vi "Data window -- tdms manage.vi"(7 "Data window action":T1, 8 "Length IN":i32, 9 "Start IN":i64, 11 "Data window IN":T2={"Start"=313333, "Length"=3333, "Channel numbers"=[0], "Channel names"=["freq", "Field"], "Group name"="p"}) -> (0 "Length OUT":i32, 1 "Start OUT":i64, 3 "Data window OUT":T2={"Start"=313333, "Length"=3333, "Channel numbers"=[0], "Channel names"=["freq", "Field"], "Group name"="p"})   [LabVIEW 2021]
uses:
  fft -- data win.ctl
  Data window -- tdms manage -- control.ctl
panel:
  # "OR"
  # "OR"
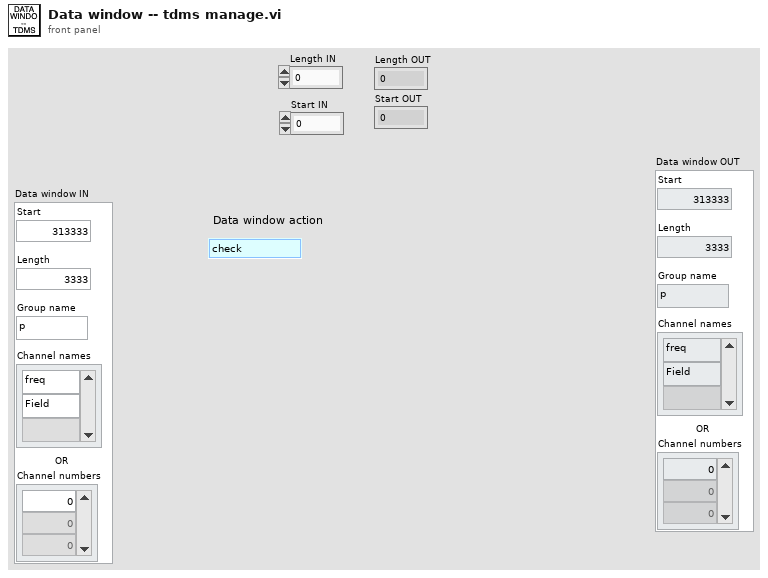
[diagram p1: front panel]
types:
  T1 = typedef "Data window -- tdms manage -- control.ctl" = enum16{"check", "set start&len", "set field channel", "set freq channel"}
  T2 = typedef "fft -- data win.ctl" = cluster{"Start":i64, "Length":i32, "Channel numbers":i64[], "Channel names":string[], "Group name":string}
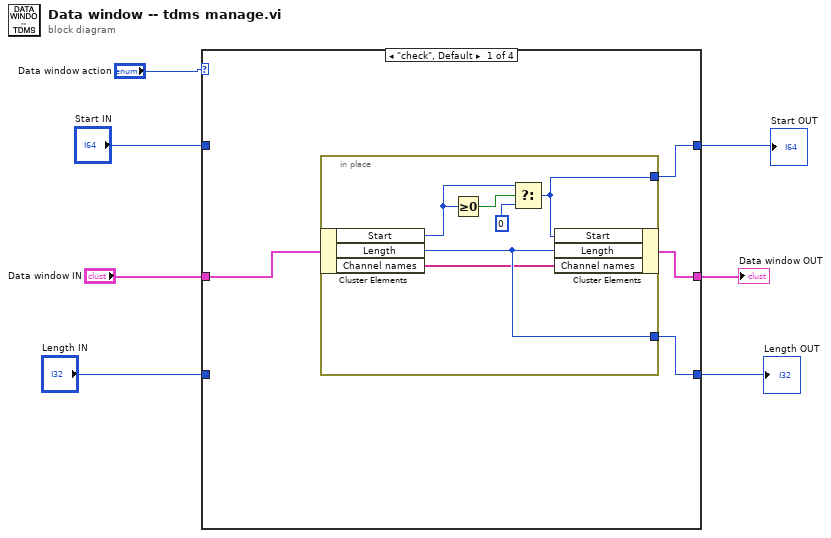
[diagram p0: block diagram]
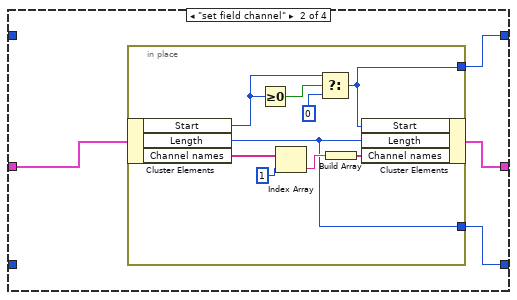
[diagram p2: hidden frame]
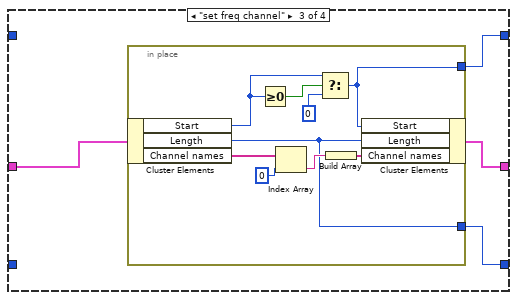
[diagram p3: hidden frame]
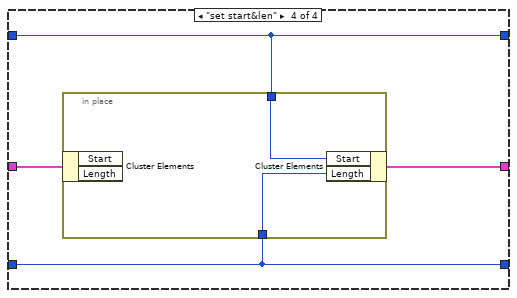
[diagram p4: hidden frame]
diagram:
  n1 = case shown="\"check\", Default" "Data window action" {
    tunnel: "Data window IN" -> [w11 w21 w34 w44]
    tunnel: [w10 w20 w33 w47] -> w5
    tunnel: [w9 w19 w32 w45] -> w4
    tunnel: [w8 w18 w31 w46] -> w3
    tunnel: "Start IN" -> [_ _ _ w46]
    tunnel: "Length IN" -> [_ _ _ w45]
    frame "check", Default {
      n2 = in-place {
        in-place-border: [w14] -> w9
        in-place-border: [w13] -> w8
        n3 = in-place-cluster #1(w11) -> ("Start"=w15:i64, "Length"=w14:i32, "Channel names"=w12:string[])
        n4 = Greater Or Equal To 0?(x=w15) -> (x >= 0?=w17:bool)
        n5 = Select(t=w15, s=w17, f=i64 0 ("Start")) -> (s? t:f=w13:i64)
        n6 = in-place-cluster #1("Start"=w13, "Length"=w14, "Channel names"=w12) -> (w10:T2)
      }
    }
    frame "set field channel" {
      n7 = in-place {
        in-place-border: [w23] -> w19
        in-place-border: [w22] -> w18
        n8 = in-place-cluster #2(w21) -> ("Start"=w24:i64, "Length"=w23:i32, "Channel names"=w28:string[])
        n9 = Greater Or Equal To 0?(x=w24) -> (x >= 0?=w30:bool)
        n10 = Index Array(array=w28, index=1) -> (element=w27:string)
        n11 = Select(t=w24, s=w30, f=i64 0 ("Start")) -> (s? t:f=w22:i64)
        n12 = Build Array(w27) -> (w26:string[])
        n13 = in-place-cluster #2("Start"=w22, "Length"=w23, "Channel names"=w26) -> (w20:T2)
      }
    }
    frame "set freq channel" {
      n14 = in-place {
        in-place-border: [w36] -> w32
        in-place-border: [w35] -> w31
        n15 = in-place-cluster #3(w34) -> ("Start"=w37:i64, "Length"=w36:i32, "Channel names"=w41:string[])
        n16 = Greater Or Equal To 0?(x=w37) -> (x >= 0?=w43:bool)
        n17 = Index Array(array=w41, index=0) -> (element=w40:string)
        n18 = Select(t=w37, s=w43, f=i64 0 ("Start")) -> (s? t:f=w35:i64)
        n19 = Build Array(w40) -> (w39:string[])
        n20 = in-place-cluster #3("Start"=w35, "Length"=w36, "Channel names"=w39) -> (w33:T2)
      }
    }
    frame "set start&len" {
      n21 = in-place {
        in-place-border: w46 -> [w49]
        in-place-border: w45 -> [w48]
        n22 = in-place-cluster #4(w44) -> ()  [unwired: 2 out]
        n23 = in-place-cluster #4("Start"=w49, "Length"=w48) -> (w47:T2)
      }
    }
  }
  "Data window OUT" <- w5
  "Length OUT" <- w4
  "Start OUT" <- w3
